vi "Send Images To PC Flip.vi"(8 "error in (no error)":errorcluster, 10 "FlipImage":bool, 11 "CameraDevRef":T1) -> ()   [LabVIEW 2015]
doc: "This VI is used to send images to the dashboard using the second enet port on the 8 slot controller. This is provided for compatibility, but is higher overhead than using the Camera MJPG approach.\n\nThis software is licensed. Open the labview\\readme\\WPI Robotics Library Open Source License.txt file for more information."
uses:
  <vilib>/Rock Robotics/WPI/Camera/WPI_CameraDevRef.ctl
  <vilib>/Rock Robotics/SystemInterfaces/NetworkCommunication/NetComm_UsageReport_ResourceType.ctl
  <vilib>/vision/NI_Vision_Development_Module.lvlib
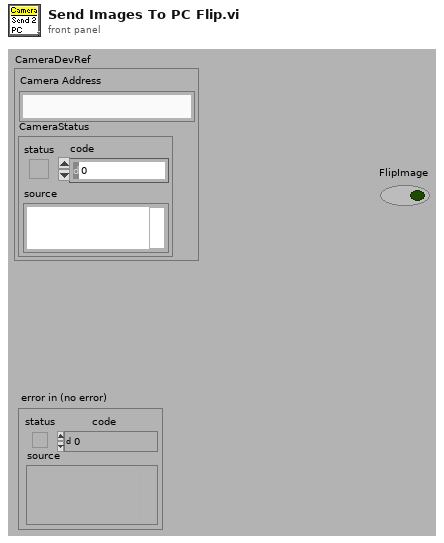
[diagram p1: front panel]
types:
  T1 = typedef "WPI_CameraDevRef.ctl" = cluster{"Camera Address":string, "CameraStatus":errorcluster}
  T2 = cluster{"fps":i32, "compression":i32, "compression 2":i32}
  T3 = typedef "NetComm_UsageReport_ResourceType.ctl" = enum8{"Controller", "Module", "Language", "CANPlugin", "Accelerometer", "ADXL345", "AnalogChannel", "AnalogTrigger", "AnalogTriggerOutput", "CANJaguar", "Compressor", "Counter", "Dashboard", "DigitalInput", "DigitalOutput", "DriverStationCIO", "DriverStationEIO", "DriverStationLCD", "Encoder", "GearTooth", "Gyro", "I2C", "Framework", "Jaguar", "Joystick", "Kinect", "KinectStick", "PIDController", "Preferences", "PWM", "Relay", "RobotDrive", "SerialPort", "Servo", "Solenoid", "SPI", "Task", "Ultrasonic", "Victor", "Button", "Command", "AxisCamera", "PCVideoServer", "SmartDashboard", "Talon", "HiTechnicColorSensor", "HiTechnicAccel", "HiTechnicCompass", "SRF08", "AnalogOutput", "Victor SP", "Talon SRX", "CAN Talon SRX", "ADXL362 Accel", "ADXRS450 Gyro", "Rev SPARK", "Mindsensors SD540", "Digital Filter"}
  T4 = enum16{"Update Mode", "Get Image", "Get Image Data"}
  T5 = typedef "Image Type" = u32
  T6 = typedef "IMAQ Image.ctl" = refnum<image>
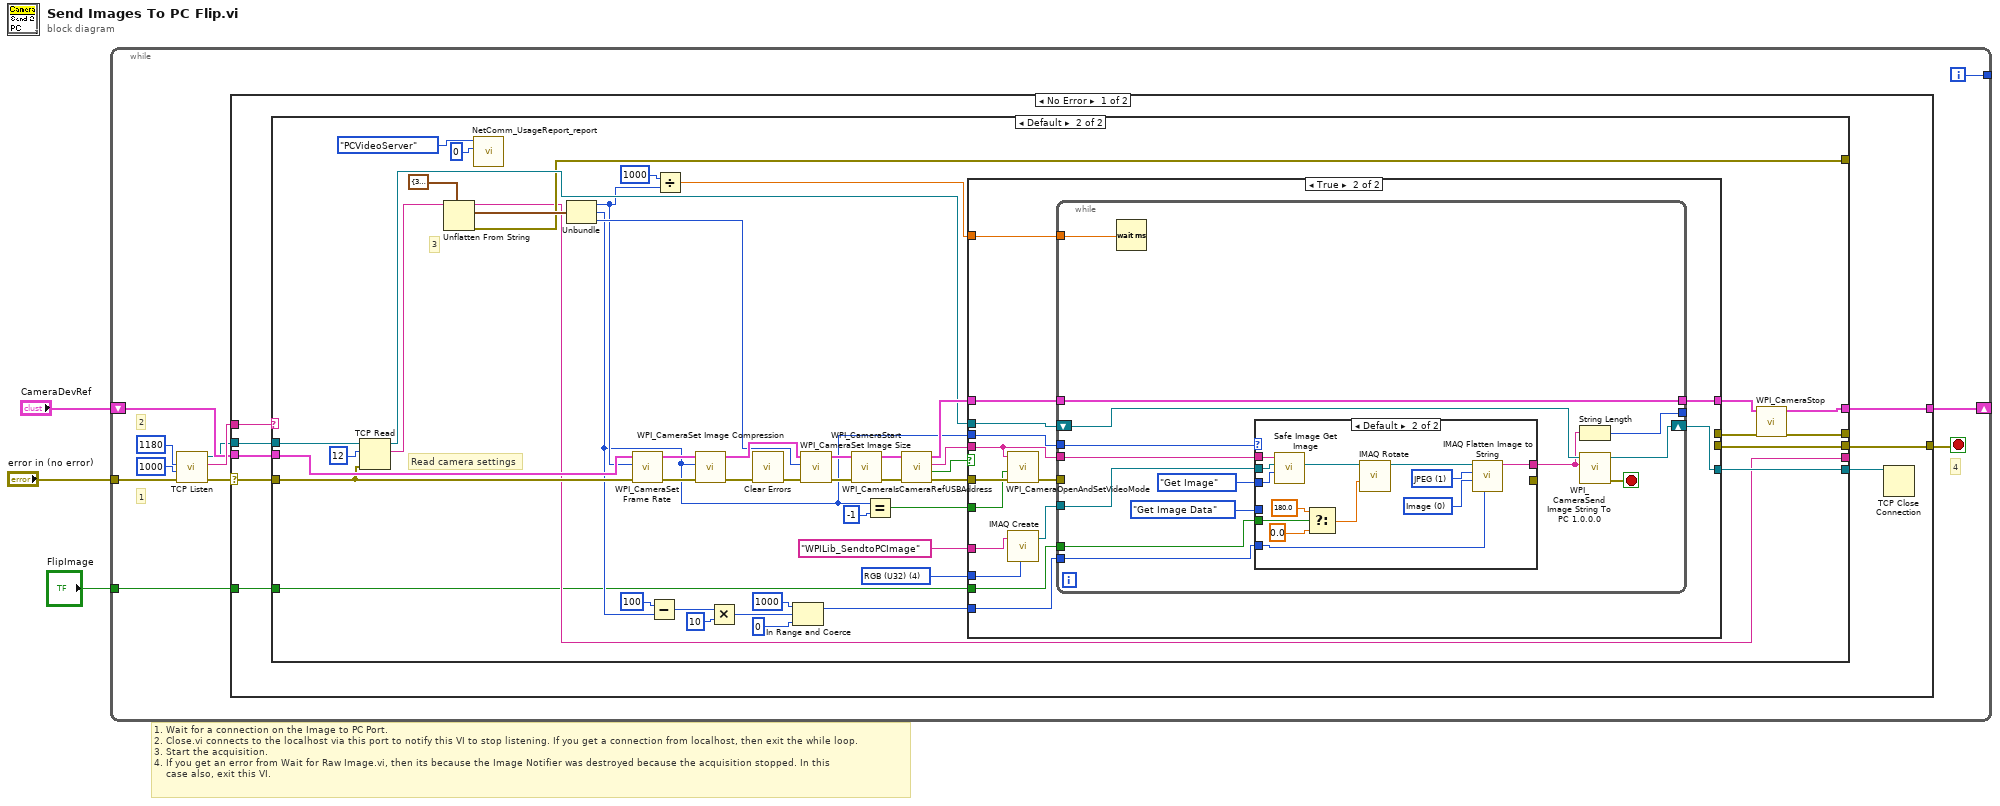
[diagram p0: block diagram]
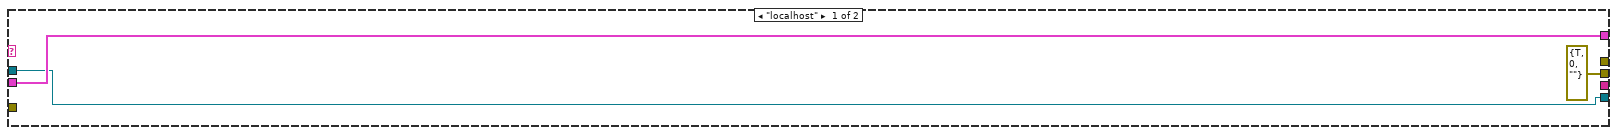
[diagram p2: hidden frame]
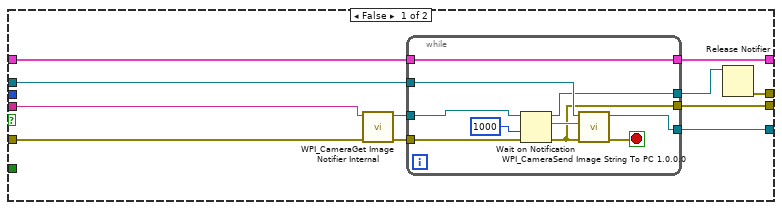
[diagram p3: hidden frame]
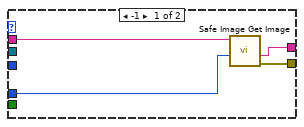
[diagram p4: hidden frame]
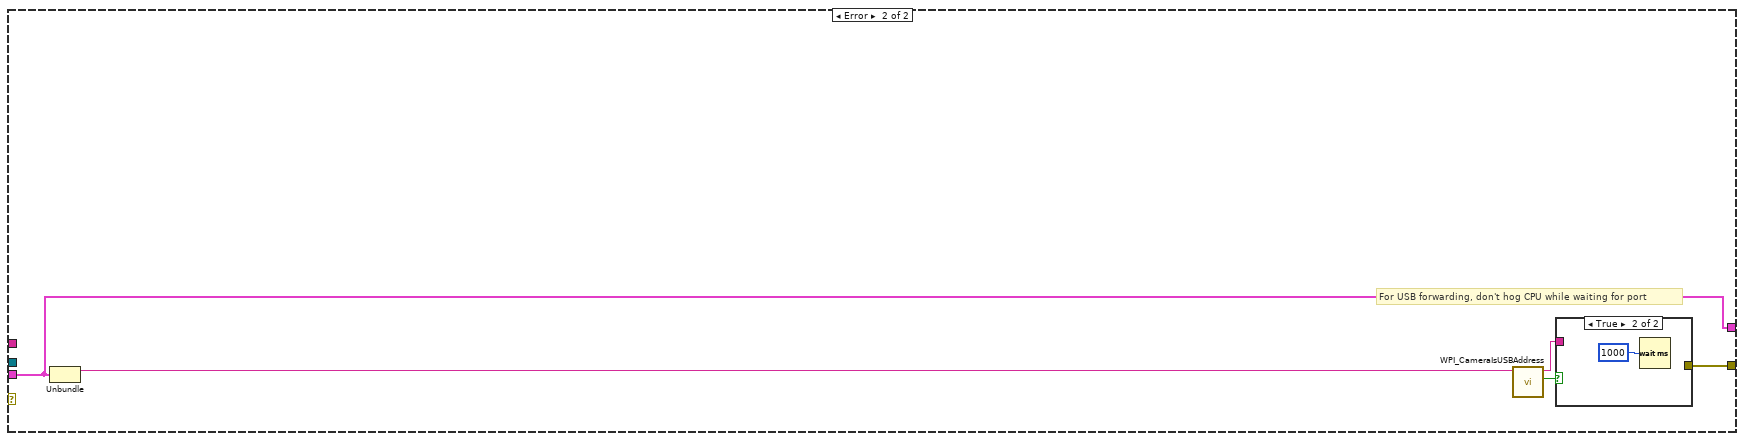
[diagram p5: hidden frame]
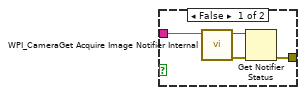
[diagram p6: hidden frame]
diagram:
  # "1. Wait for a connection on the Image to PC Port.\n2. Close.vi connects to the localhost via this port to notify this VI to stop listening. If you get a connection from localhost, then exit the while loop.\n3. Start the acquisition.\n4. If you get an error from Wait for Raw Image.vi, then its because the Image Notifier was destroyed because the acquisition stopped. In this\n    case also, exit this VI."
  n1 = while {
    tunnel: "error in (no error)" -> [w11]
    shift-right: [w14] -> _
    shift-left: "CameraDevRef" -> [w12]
    tunnel: [w5] -> _
    tunnel: "FlipImage" -> [w4]
    i -> [w5]
    stop <- w9 stop-if-true
    # "4"
    # "1"
    # "2"
    n2 = call <vilib>:"TCP Listen.vi"("error in (no error)"=w11, "timeout ms (wait forever: -1)"=u16 1000 ("port"), "port"=u16 1180) -> ("error out"=w7:errorcluster, "remote address"=w13:string, "connection ID"=w10:refnum<k5>)  [unwired: 1 in, 5 out]
    n3 = case shown="No Error" w7 {
      selector: w7 -> [w16 _]
      tunnel: [w22 w144] -> w14
      tunnel: w13 -> [w21 _]
      tunnel: w12 -> [w20 w144]
      tunnel: w10 -> [w19 _]
      tunnel: [w18 w145] -> w9
      tunnel: w4 -> [w15 _]
      frame No Error {
        n4 = case shown="Default" w21 {
          tunnel: [w25 w71] -> w22
          tunnel: w20 -> [w25 w53]
          tunnel: w16 -> [_ w49]
          tunnel: w19 -> [w23 w57]
          tunnel: [errorcluster {"status"=TRUE, "code"=0, "source"=""} ("error out 2") w73] -> w18
          tunnel: [w23 w72] -> w17
          tunnel: [_ w70] -> _
          tunnel: [_ w28] -> _
          tunnel: [_ w27] -> _
          tunnel: w15 -> [_ w26]
          frame "localhost" {
          }
          frame Default {
            w64 = T5 4 items=["Grayscale (U8)", "Grayscale (I16)", "Grayscale (SGL)", "Complex (CSG)", "RGB (U32)", "HSL (U32)", "RGB (U64)", "Grayscale (U16)"] ("Image Type")
            # "Read camera settings"
            # "3"
            n5 = TCP Read(connection ID=w57, bytes to read=12, error in (no error)=w49) -> (connection ID out=w56:refnum<k5>, data out=w54:string)  [unwired: 2 in, 1 out]
            n6 = Unflatten From String(type=T2 {"fps"=30, "compression"=32, "compression 2"=32} ("Camera Settings"), binary string=w54) -> (rest of the binary string=w27:string, value=w46:T2, error out=w28:errorcluster)  [unwired: 3 in]
            n7 = call <vilib>:"NetComm_UsageReport_report.vi"("Instance Number"=u8 0, "Resource Type"=NetComm_UsageReport_ResourceType."PCVideoServer") -> ()  [unwired: 10 in]
            n8 = Unbundle(w46) -> ("fps"=w43:i32, "compression"=w32:i32, "compression 2"=w45:i32)
            n9 = call <vilib>:"WPI_CameraSet Frame Rate.vi"("error in (no error)"=w49, "Frame Rate (fps)"=w43, "CameraDevRef"=w53) -> ("error out"=w48:errorcluster, "CameraDevRef Out"=w52:T1)  [unwired: 7 in]
            n10 = Subtract(x=100, y=w32) -> (x-y=w37:i32)
            n11 = Divide(x=u16 1000 ("port"), y=w43) -> (x/y=w42:dbl)
            n12 = call <vilib>:"WPI_CameraSet Image Compression.vi"("error in (no error)"=w48, "Compression"=w32, "CameraDevRef"=w52) -> ("error out"=w30:errorcluster, "CameraDevRef Out"=w51:T1)  [unwired: 7 in]
            n13 = Multiply(x=w37, y=10) -> (x*y=w39:i32)
            n14 = call <vilib>:"Clear Errors.vi"("error in (no error)"=w30) -> ("error out"=w29:errorcluster)  [unwired: 5 in, 1 out]
            n15 = In Range and Coerce(upper limit=1000, x=w39, lower limit=0) -> (coerced(x)=w35:i32)  [unwired: 1 out]
            n16 = call <vilib>:"WPI_CameraSet Image Size.vi"("error in (no error)"=w29, "Image Size"=w45, "CameraDevRef"=w51) -> ("error out"=w47:errorcluster, "CameraDevRef Out"=w50:T1)  [unwired: 7 in]
            n17 = call <vilib>:"WPI_CameraStart.vi"("error in (no error)"=w47, "CameraDevRef"=w50) -> ("error out"=w61:errorcluster, "CameraDevRef"=w59:T1)  [unwired: 8 out]
            n18 = Equal?(x=w32, y=-1) -> (x = y?=w31:bool)
            n19 = call <vilib>:"WPI_CameraIsCameraRefUSBAddress.vi"("error in (no error)"=w61, "CameraDevRef"=w59) -> ("error out"=w60:errorcluster, "USB?"=w62:bool, "Camera Address Out"=w63:string, "CameraDevRef out"=w58:T1)  [unwired: 6 in]
            n20 = case shown="True" w62 {
              tunnel: w56 -> [w84 w109]
              tunnel: [w83 _] -> w73
              tunnel: [w82 w108] -> w72
              tunnel: w60 -> [w81 w99]
              tunnel: w63 -> [w79 w98]
              tunnel: [w78 w103] -> w69
              tunnel: w58 -> [w77 w104]
              tunnel: [w75 _] -> w68
              tunnel: "WPILib_SendtoPCImage" -> [_ w106]
              tunnel: w64 -> [_ w105]
              tunnel: w35 -> [_ w102]
              tunnel: w42 -> [_ w101]
              tunnel: w32 -> [_ w100]
              tunnel: w31 -> [_ w96]
              tunnel: w26 -> [_ w95]
              frame False {
                n21 = call <vilib>:"WPI_CameraGet Image Notifier Internal.vi"("error in (no error)"=w81, "Camera Address"=w79) -> ("error out"=w80:errorcluster, "Image Notifier"=w76:refnum<notifier>)  [unwired: 8 out]
                n22 = while {
                  tunnel: w80 -> [w90]
                  tunnel: w84 -> [w94]
                  tunnel: [w87] -> w83
                  tunnel: [w92] -> w82
                  tunnel: [w91] -> w78
                  tunnel: w77 -> [w91]
                  tunnel: w76 -> [w89]
                  tunnel: [w85] -> w74
                  stop <- w93 stop-if-true
                  n23 = Wait on Notification(notifier=w89, timeout in ms (-1)=1000 ("Timeout in ms (-1)"), error in (no error)=w90) -> (notifier out=w85:refnum<notifier>, notification=w88:string, error out=w87:errorcluster)  [unwired: 2 out]
                  n24 = call <vilib>:"WPI_CameraSend Image String To PC 1.0.0.0.vi"("error in (no error)"=w87, "String"=w88, "TCP Connection ID"=w94) -> ("error out"=w93:errorcluster, "TCP Connection ID out"=w92:refnum<k5>)  [unwired: 7 out]
                }
                n25 = Release Notifier(notifier=w74) -> (error out=w75:errorcluster)  [unwired: 1 in, 3 out]
              }
              frame True {
                n26 = call <vilib>:"WPI_CameraOpenAndSetVideoMode.vi"("error in (no error)"=w99, "USB JPEG"=w96, "Camera Address Out"=w98) -> ("error out"=w97:errorcluster)  [unwired: 8 in]
                n27 = call "IMAQ Create"("Image Name"=w106, "Image Type"=w105) -> ("New Image"=w107:T6)  [unwired: 3 in, 1 out]
                n28 = while {
                  tunnel: w98 -> [w122]
                  shift-right: [w123] -> w108
                  shift-left: w109 -> [w116]
                  tunnel: w107 -> [w121]
                  tunnel: [w119] -> w103
                  tunnel: w104 -> [w119]
                  tunnel: w102 -> [w118]
                  tunnel: w101 -> [w117]
                  tunnel: [w114] -> _
                  tunnel: w100 -> [w113]
                  tunnel: w97 -> [_]
                  tunnel: w95 -> [w110]
                  stop <- w120 stop-if-true
                  n29 = Wait (ms)(milliseconds to wait=w117) -> ()  [unwired: 1 out]
                  n30 = case shown="Default" w113 {
                    tunnel: [w126 w140] -> w115
                    tunnel: w122 -> [w127 w136]
                    tunnel: w121 -> [_ w135]
                    tunnel: w118 -> [_ w137]
                    tunnel: [w125 _] -> _
                    tunnel: T4."Get Image Data" ("Operation") -> [w124 _]
                    tunnel: T4."Get Image" ("Operation") -> [_ w132]
                    tunnel: w110 -> [_ w128]
                    frame -1 {
                      n31 = call <vilib>:"Safe Image Get Image.vi"("Operation"=w124, "Session In"=w127) -> ("error out"=w125:errorcluster, "Image Data String"=w126:string)  [unwired: 6 in, 2 out]
                    }
                    frame Default {
                      w138 = 0 items=["Image", "Image and Vision Info", "Reference to Image"] ("Type of Flatten (Image and Vision Info)")
                      w139 = 1 items=["None", "JPEG", "PACKED BINARY"] ("Compression (None)")
                      n32 = call <vilib>:"Safe Image Get Image.vi"("Operation"=w132, "Image In"=w135, "Session In"=w136) -> ("Image Out"=w134:T6)  [unwired: 5 in, 3 out]
                      n33 = Select(t=sgl 180.0, s=w128, f=sgl 0.0) -> (s? t:f=w131:sgl)
                      n34 = call "IMAQ Rotate"("Angle (degrees)"=w131, "Image Src"=w134) -> ("Image Dst Out"=w133:T6)  [unwired: 8 in, 1 out]
                      n35 = call "IMAQ Flatten Image to String"("Quality (750)"=w137, "Type of Flatten (Image and Vision Info)"=w138, "Compression (None)"=w139, "Image"=w133) -> ("Data String"=w140:string)  [unwired: 6 in, 1 out]
                    }
                  }
                  n36 = String Length(string=w115) -> (length=w114:i32)
                  n37 = call <vilib>:"WPI_CameraSend Image String To PC 1.0.0.0.vi"("String"=w115, "TCP Connection ID"=w116) -> ("error out"=w120:errorcluster, "TCP Connection ID out"=w123:refnum<k5>)  [unwired: 1 in, 7 out]
                }
              }
            }
            n38 = call <vilib>:"WPI_CameraStop.vi"("error in (no error)"=w68, "CameraDevRef"=w69) -> ("error out"=w70:errorcluster, "CameraDevRef"=w71:T1)  [unwired: 8 out]
          }
        }
        n39 = TCP Close Connection(connection ID=w17) -> ()  [unwired: 1 in, 3 out]
      }
      frame Error {
        # "For USB forwarding, don't hog CPU while waiting for port"
        n40 = Unbundle(w144) -> ("Camera Address"=w143:string)  [unwired: 1 out]
        n41 = call <vilib>:"WPI_CameraIsUSBAddress.vi"("Camera Address In"=w143) -> ("USB?"=w141:bool, "Camera Address Out"=w142:string)  [unwired: 8 in, 1 out]
        n42 = case shown="True" w141 {
          tunnel: [w149 _] -> w145
          tunnel: w142 -> [w146 _]
          frame False {
            n43 = call <vilib>:"WPI_CameraGet Acquire Image Notifier Internal.vi"("Camera Address"=w146) -> ("error out"=w147:errorcluster, "Acquire Image Notifier"=w148:refnum<notifier>)  [unwired: 1 in, 8 out]
            n44 = Get Notifier Status(notifier=w148, error in (no error)=w147) -> (error out=w149:errorcluster)  [unwired: 4 out]
          }
          frame True {
            n45 = Wait (ms)(milliseconds to wait=u32 1000) -> ()  [unwired: 1 out]
          }
        }
      }
    }
  }
